vi "writecoefficientsettings.vi"(1 "Path":path, 2 "?":T1, 5 "error in (no error)":errorcluster) -> (6 "Path 2":path, 8 "error out":errorcluster)   [LabVIEW 2012]
uses:
  <vilib>/Utility/config.llb/Write Key (Double).vi
  <vilib>/Utility/config.llb/NI_LVConfig.lvlib
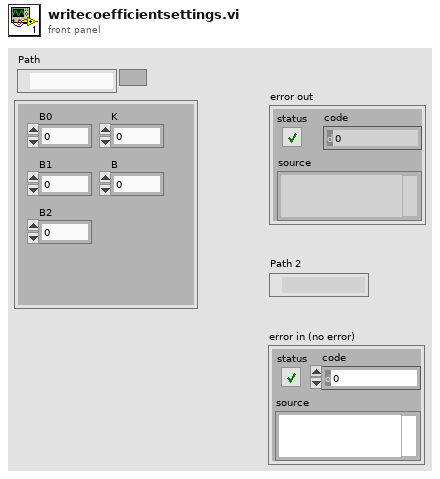
[diagram p1: front panel]
types:
  T1 = cluster{"B0":dbl, "B1":dbl, "B2":dbl, "K":dbl, "B":dbl}
  T2 = typedef "NI_LVConfig.lvlib/Config Data RefNum.ctl" = refnum<k1>
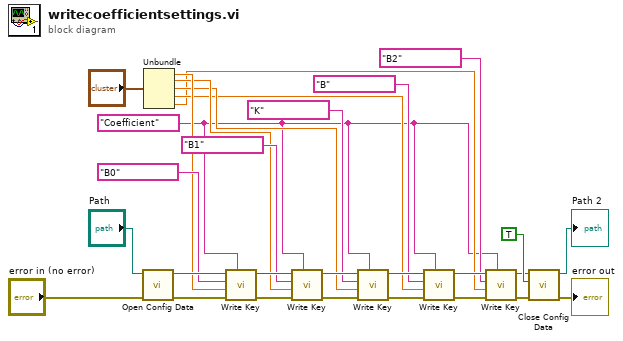
[diagram p0: block diagram]
diagram:
  w2 = "Coefficient"
  n1 = call <vilib>:"Open Config Data.vi"("error in (no error)"="error in (no error)", "configuration file path"="Path") -> ("error out"=w23:errorcluster, "refnum"=w28:T2)  [unwired: 7 in, 1 out]
  n2 = Unbundle("?") -> ("B0"=w11:dbl, "B1"=w10:dbl, "B2"=w9:dbl, "K"=w8:dbl, "B"=w7:dbl)
  n3 = call-poly <vilib>:"Write Key.vi"("section"=w2, "error in (no error)"=w23, "value"=w11, "key"="B0", "refnum"=w28) -> ("error out"=w22:errorcluster, "refnum out"=w27:T2)  [unwired: 4 in, 1 out]
  n4 = call-poly <vilib>:"Write Key.vi"("section"=w2, "error in (no error)"=w22, "value"=w10, "key"="B1", "refnum"=w27) -> ("error out"=w21:errorcluster, "refnum out"=w26:T2)  [unwired: 4 in, 1 out]
  n5 = call-poly <vilib>:"Write Key.vi"("section"=w2, "error in (no error)"=w21, "value"=w9, "key"="K", "refnum"=w26) -> ("error out"=w20:errorcluster, "refnum out"=w25:T2)  [unwired: 4 in, 1 out]
  n6 = call-poly <vilib>:"Write Key.vi"("section"=w2, "error in (no error)"=w20, "value"=w8, "key"="B", "refnum"=w25) -> ("error out"=w19:errorcluster, "refnum out"=w24:T2)  [unwired: 4 in, 1 out]
  n7 = call-poly <vilib>:"Write Key.vi"("section"=w2, "error in (no error)"=w19, "value"=w7, "key"="B2", "refnum"=w24) -> ("error out"=w3:errorcluster, "refnum out"=w4:T2)  [unwired: 4 in, 1 out]
  n8 = call <vilib>:"Close Config Data.vi"("error in (no error)"=w3, "write file if changed (T)"=TRUE, "refnum"=w4) -> ("error out"=→"error out":errorcluster, "file path"=→"Path 2":path)  [unwired: 7 in]
